vi "Medidor de tanque.vi"() -> ()   [LabVIEW 2017]
panel:
  in  "stop":bool
  out "Lleno":bool
  out "Normal":bool
  out "Vacio":bool
  out "?":dbl(slide) scale=0.0..100.0
  in  "Nivel":dbl
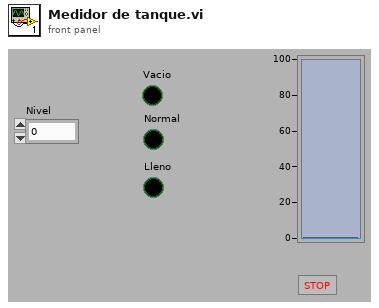
[diagram p1: front panel]
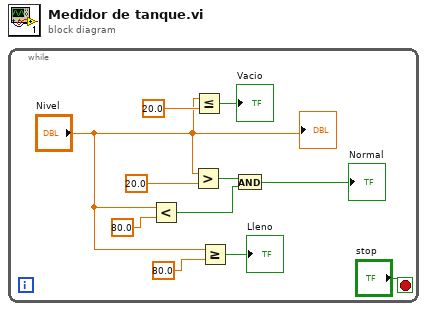
[diagram p0: block diagram]
diagram:
  n1 = while {
    stop <- "stop" stop-if-true
    n2 = Less?(x="Nivel", y=80.0 ("Numeric 2")) -> (x < y?=w6:bool)
    n3 = Greater?(x="Nivel", y=20.0 ("Numeric 2")) -> (0:w7:bool)
    n4 = Less Or Equal?(x="Nivel", y=20.0 ("Numeric 2")) -> (x <= y?=→"Vacio":bool)
    n5 = Greater Or Equal?(x="Nivel", y=80.0 ("Numeric 2")) -> (x >= y?=→"Lleno":bool)
    n6 = And(x=w7, y=w6) -> (x .and. y?=→"Normal":bool)
    "?" <- "Nivel"
  }
